vi "main.vi"() -> ()   [LabVIEW 2019]
panel:
  out "String":string="a"
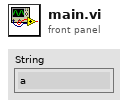
[diagram p1: front panel]
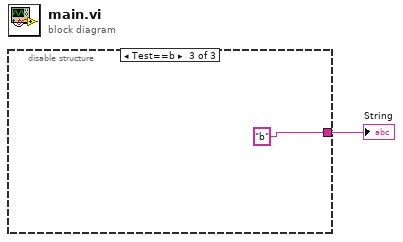
[diagram p0: block diagram]
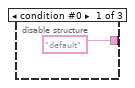
[diagram p2: hidden frame]
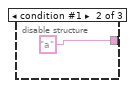
[diagram p3: hidden frame]
diagram:
  n1 = disable-structure shown="Test==b" {
    disable-tunnel: ["default" "a" "b"] -> w1
    frame condition #0 {
    }
    frame condition #1 {
    }
    frame condition #2 (active) {
    }
  }
  "String" <- w1
